vi "adaptationImpedance.vi"(7 "decimal / hexa":bool, 8 "error in":errorcluster, 10 "adress":string, 11 "value (decimal":u8=255) -> (0 "error out":errorcluster)   [LabVIEW 2017]
uses:
  <vilib>/FIME/_Switcher_internal_deps/USB_I2C_adaptor_ftdi.dll
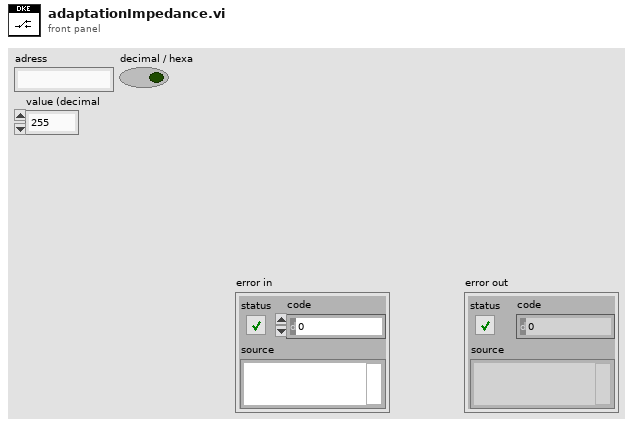
[diagram p1: front panel]
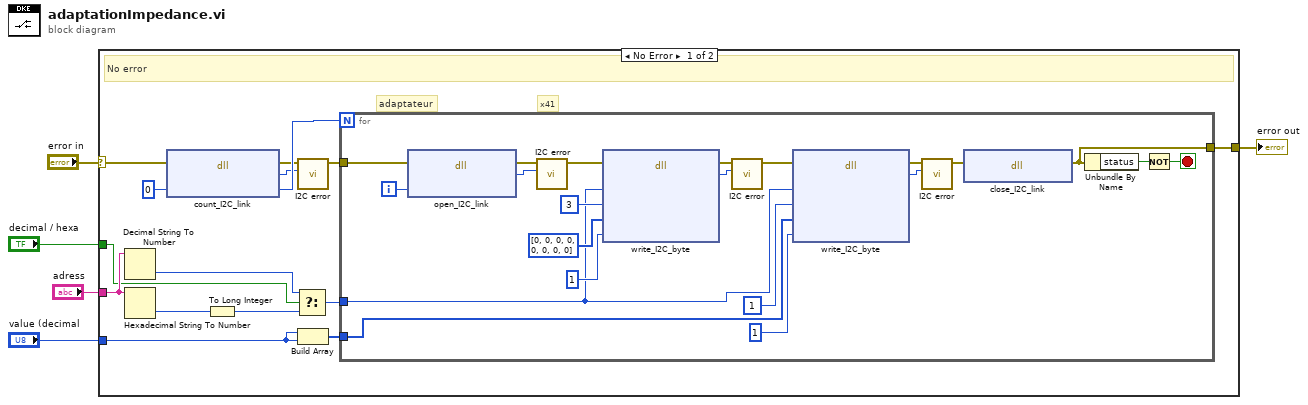
[diagram p0: block diagram]
diagram:
  n1 = case shown="No Error" "error in" {
    selector: "error in" -> [w15 w42]
    tunnel: [w14 w42] -> w5
    tunnel: "adress" -> [w9 _]
    tunnel: "value (decimal" -> [w7 _]
    tunnel: "decimal / hexa" -> [w6 _]
    frame No Error {
      # "adaptateur"
      # "x41"
      # "No error"
      n2 = Decimal String To Number(string=w9) -> (number=w13:i32)  [unwired: 2 in, 1 out]
      n3 = Hexadecimal String To Number(string=w9) -> (number=w11:u32)  [unwired: 2 in, 1 out]
      n4 = dll-call lib="C:/Program Files (x86)/National Instruments/LabVIEW 2017/vi.lib/FIME/_Switcher_internal_deps/USB_I2C_adaptor_ftdi.dll" fn="count_I2C_link" label="I2C"(error in=w15, "channels_p"=0) -> (error out=w18:errorcluster, "return type"=w16:i32, "channels_p"=w20:i32)  [unwired: 2 in, 1 out]
      n5 = To Long Integer(number=w11) -> (32bit integer=w10:i32)
      n6 = Select(t=w13, s=w6, f=w10) -> (s? t:f=w12:i32)
      n7 = call "I2C error.vi"("return"=w16, "error in"=w18) -> ("error out"=w17:errorcluster)  [unwired: 4 in, 5 out]
      n8 = Build Array(w7, w7) -> (w8:u8[])
      n9 = for {
        N: w20 -> [_]
        tunnel: w17 -> [w41]
        tunnel: [w31] -> w14
        tunnel: w12 -> [w22]
        tunnel: w8 -> [w21]
        i -> [w24]
        stop <- w37 stop-if-true
        n10 = dll-call lib="C:/Program Files (x86)/National Instruments/LabVIEW 2017/vi.lib/FIME/_Switcher_internal_deps/USB_I2C_adaptor_ftdi.dll" fn="open_I2C_link" label="I2C"(error in=w41, "channel"=w24) -> (error out=w40:errorcluster, "return type"=w39:i32)  [unwired: 3 in, 1 out]
        n11 = call "I2C error.vi"("return"=w39, "error in"=w40) -> ("error out"=w32:errorcluster)  [unwired: 4 in, 5 out]
        n12 = dll-call lib="C:/Program Files (x86)/National Instruments/LabVIEW 2017/vi.lib/FIME/_Switcher_internal_deps/USB_I2C_adaptor_ftdi.dll" fn="write_I2C_byte" label="I2C"(error in=w32, "slaveAddress"=w22, "registerAddress"=u8 3 ("element"), "data"=u8[] [0, 0, 0, 0, 0, 0, 0, 0], "size"=u8 1) -> (error out=w33:errorcluster, "return type"=w36:i32)  [unwired: 5 in, 2 out]
        n13 = call "I2C error.vi"("return"=w36, "error in"=w33) -> ("error out"=w23:errorcluster)  [unwired: 4 in, 5 out]
        n14 = dll-call lib="C:/Program Files (x86)/National Instruments/LabVIEW 2017/vi.lib/FIME/_Switcher_internal_deps/USB_I2C_adaptor_ftdi.dll" fn="write_I2C_byte" label="I2C"(error in=w23, "slaveAddress"=w22, "registerAddress"=u8 1 ("element"), "data"=w21, "size"=u8 1) -> (error out=w26:errorcluster, "return type"=w25:i32)  [unwired: 5 in, 2 out]
        n15 = call "I2C error.vi"("return"=w25, "error in"=w26) -> ("error out"=w27:errorcluster)  [unwired: 4 in, 5 out]
        n16 = dll-call lib="C:/Program Files (x86)/National Instruments/LabVIEW 2017/vi.lib/FIME/_Switcher_internal_deps/USB_I2C_adaptor_ftdi.dll" fn="close_I2C_link" label="I2C"(error in=w27) -> (error out=w31:errorcluster)  [unwired: 2 in, 2 out]
        n17 = Unbundle By Name(w31) -> ("status"=w38:bool)
        n18 = Not(x=w38) -> (.not. x?=w37:bool)
      }
    }
    frame Error {
      # "Error"
    }
  }
  "error out" <- w5
